vi "DetectLineColor.vi"(7 "Port/MUX":T1 {"Port" items=["Port 1", "Port 2", "Port 3", "Port 4"]; "MUX Port" items=["No MUX", "MUX 1", "MUX 2", "MUX 3", "MUX 4"]}, 11 "NXT In":T3) -> (1 "Detected Line?":bool, 3 "NXT Out":T3 caption="NXT", 4 "Color":string="Black")   [LabVIEW 2012]
uses:
  <vilib>/NXT/Subs/LVHSConnector.ctl
  <vilib>/NXT/LegoClasses/BrickReference/BrickReference.lvclass
  <vilib>/NXT/HiTechnic/HiTechnic Controls/HiTechnic Port.ctl
  <vilib>/NXT/Block Support/NXT_InputPort.ctl
  <vilib>/NXT/HiTechnic/HiTechnic SubVIs/HiTechnic Color Sensor Active Color.vi
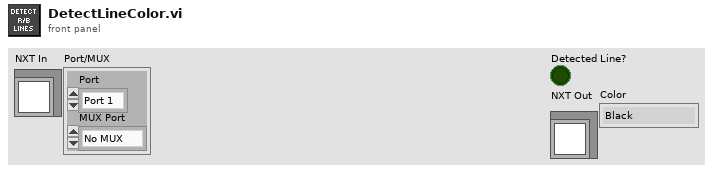
[diagram p1: front panel]
types:
  T1 = typedef "HiTechnic Port.ctl" = cluster{"Port":T2, "MUX Port":u8}
  T2 = typedef "NXT_InputPort.ctl" = u8
  T3 = typedef "LVHSConnector.ctl" = refnum<class "BrickReference.lvclass">
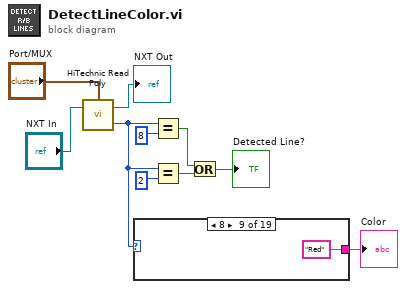
[diagram p0: block diagram]
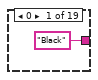
[diagram p2: hidden frame]
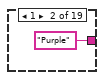
[diagram p3: hidden frame]
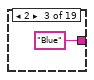
[diagram p4: hidden frame]
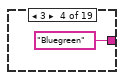
[diagram p5: hidden frame]
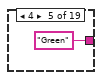
[diagram p6: hidden frame]
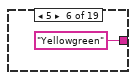
[diagram p7: hidden frame]
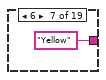
[diagram p8: hidden frame]
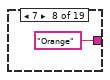
[diagram p9: hidden frame]
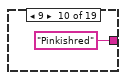
[diagram p10: hidden frame]
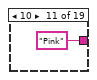
[diagram p11: hidden frame]
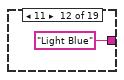
[diagram p12: hidden frame]
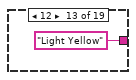
[diagram p13: hidden frame]
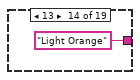
[diagram p14: hidden frame]
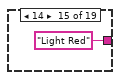
[diagram p15: hidden frame]
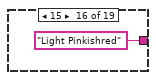
[diagram p16: hidden frame]
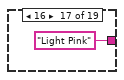
[diagram p17: hidden frame]
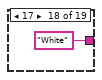
[diagram p18: hidden frame]
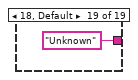
[diagram p19: hidden frame]
diagram:
  n1 = call-poly <vilib>:"HiTechnic Read Poly.vi"("NXT"="NXT In", "Port/MUX"="Port/MUX") -> ("Color Number"=w7:i32, "NXT"=→"NXT Out":T3)  [unwired: 1 in]
  n2 = case shown="8" w7 {
    tunnel: ["Black" "Purple" "Blue" "Bluegreen" "Green" "Yellowgreen" "Yellow" "Orange" "Red" "Pinkishred" "Pink" "Light Blue" "Light Yellow" "Light Orange" "Light Red" "Light Pinkishred" "Light Pink" "White" "Unknown"] -> w8
    frame 0 {
    }
    frame 1 {
    }
    frame 2 {
    }
    frame 3 {
    }
    frame 4 {
    }
    frame 5 {
    }
    frame 6 {
    }
    frame 7 {
    }
    frame 8 {
    }
    frame 9 {
    }
    frame 10 {
    }
    frame 11 {
    }
    frame 12 {
    }
    frame 13 {
    }
    frame 14 {
    }
    frame 15 {
    }
    frame 16 {
    }
    frame 17 {
    }
    frame 18, Default {
    }
  }
  "Color" <- w8
  n3 = Equal?(x=w7, y=8) -> (x = y?=w10:bool)
  n4 = Equal?(x=w7, y=2) -> (x = y?=w9:bool)
  n5 = Or(x=w10, y=w9) -> (x .or. y?=→"Detected Line?":bool)
